vi "frontEnd.vi"(8 "error in (no error)":errorcluster, 11 "ScriptEditorV2 in":refnum<class "ScriptEditorV2.lvclass">) -> (0 "error out":errorcluster, 3 "ScriptEditorV2 out":refnum<class "ScriptEditorV2.lvclass">)   [LabVIEW 2009, in "Views.lvlib" / "ScriptEditor.lvlib" / "ScriptEditorV2.lvclass"]
uses:
  ScriptEditorV2.lvclass
  ScriptEditorV2.lvclass/ScriptEditorV2.ctl
  ScriptEdEvents/ScriptEdEvents.lvclass
  Tools/DatabaseHelpers.lvlib
panel:
  in  "Delete Event":bool
  in  "highlightChannel":bool
  in  "open":bool
  in  "saveAs":bool
  in  "save":bool
  in  "Script Information":string
  out "Multicolumn Listbox":i32[](listbox)
  # "Open"
  # "save"
  # "saveAs"
  # "Highlight"
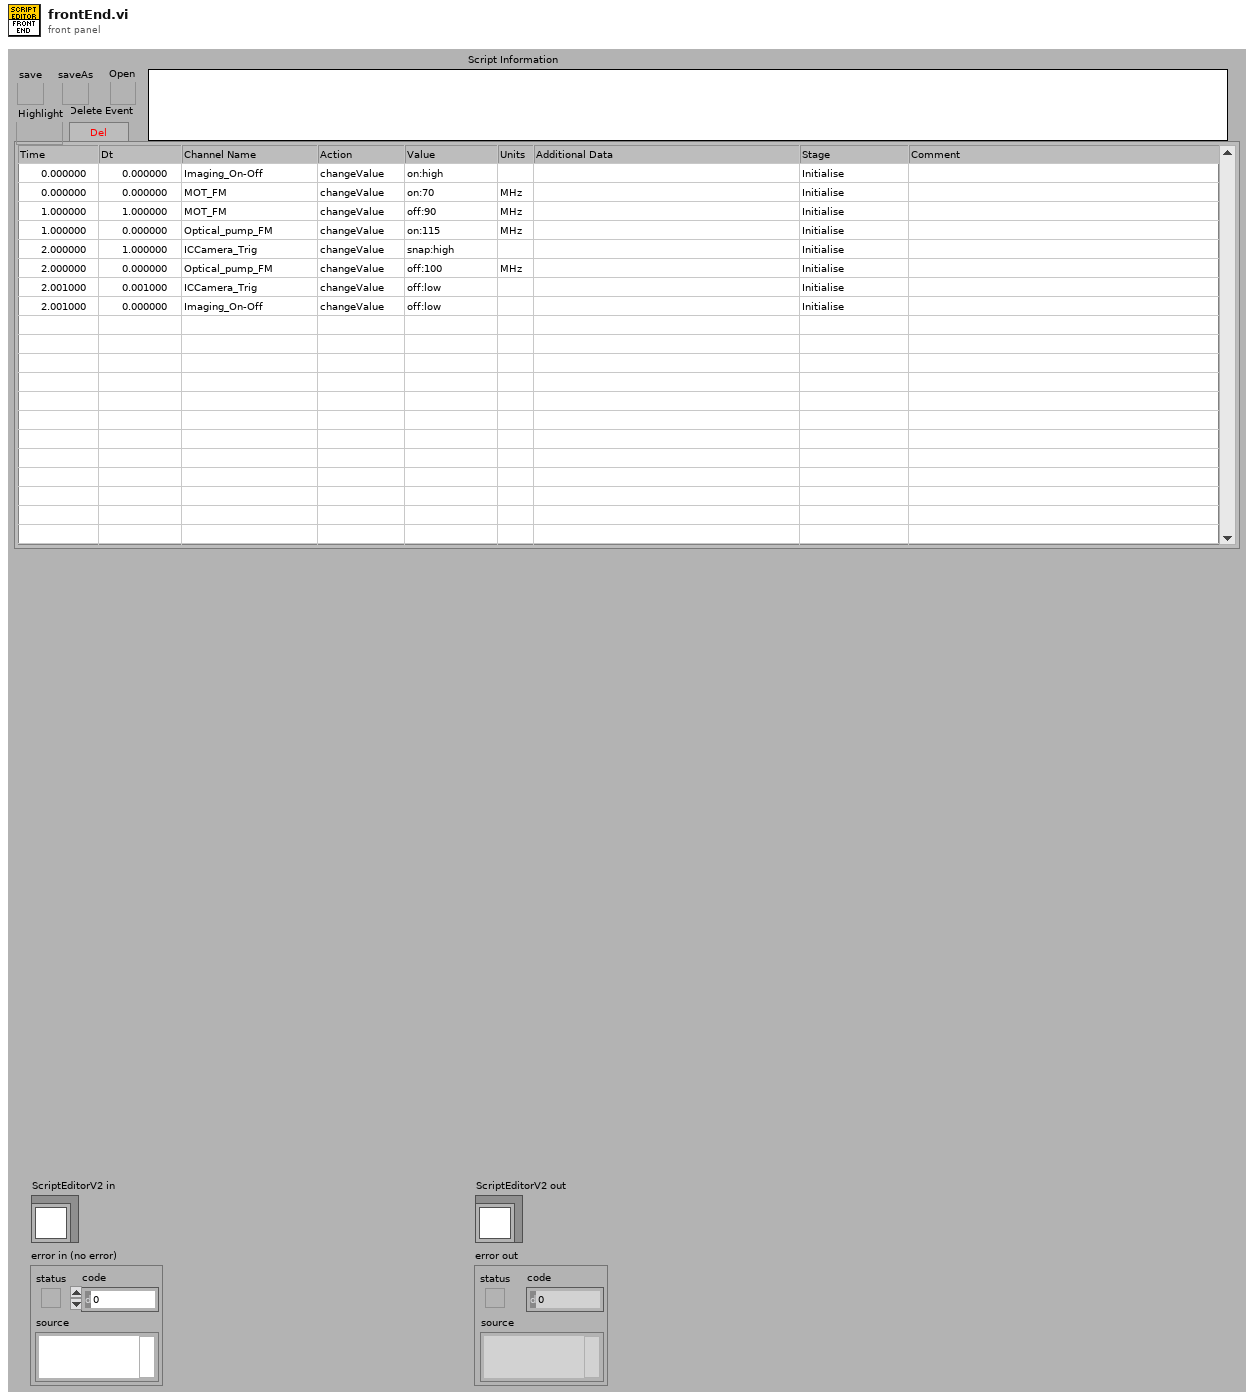
[diagram p1: front panel]
types:
  T1 = typedef "LVPoint32TypeDef.ctl" = cluster{"Horizontal":i32, "Vertical":i32}
  T2 = typedef "LVRowAndColumnTypeDef.ctl" = cluster{"Row":i32, "Column":i32}
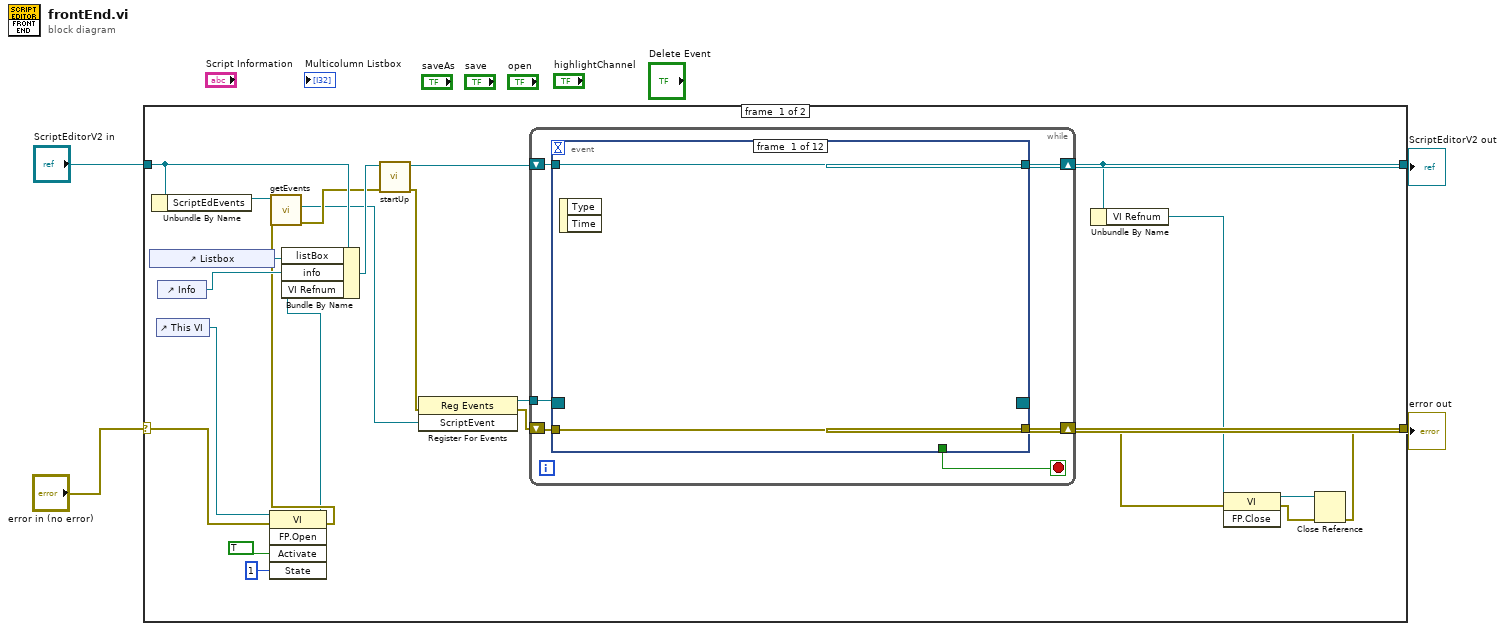
[diagram p0: block diagram]
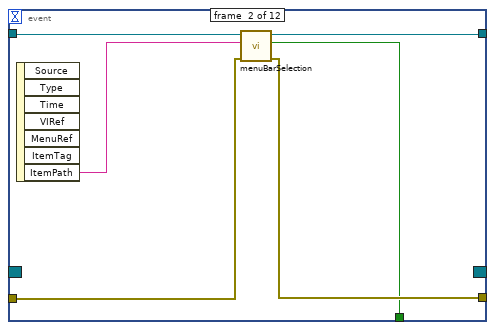
[diagram p2: hidden frame]
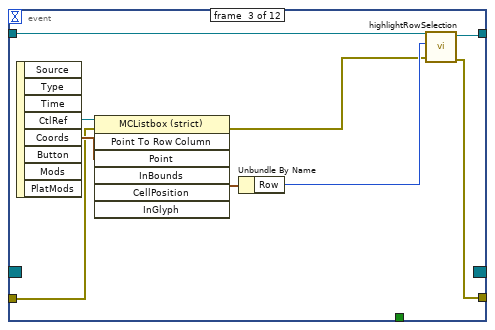
[diagram p3: hidden frame]
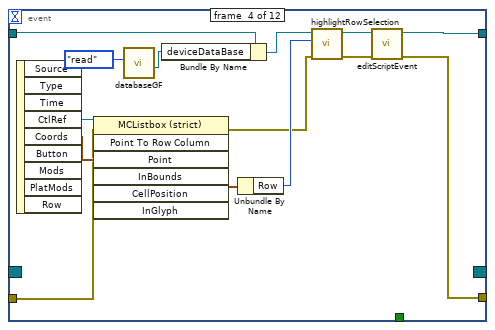
[diagram p4: hidden frame]
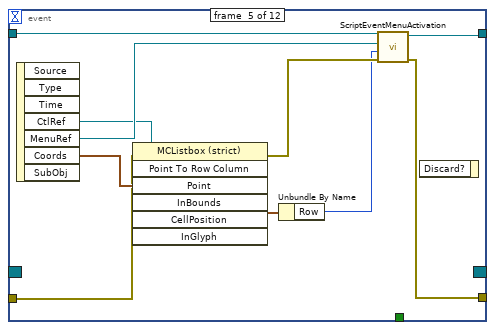
[diagram p5: hidden frame]
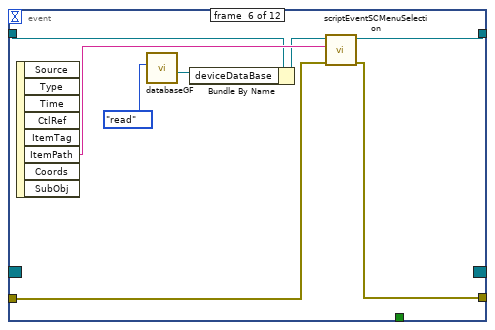
[diagram p6: hidden frame]
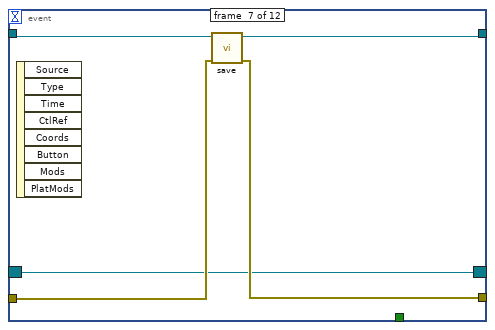
[diagram p7: hidden frame]
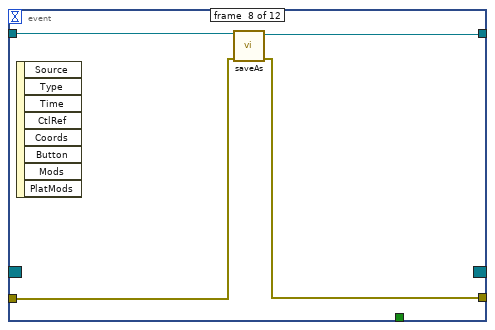
[diagram p8: hidden frame]
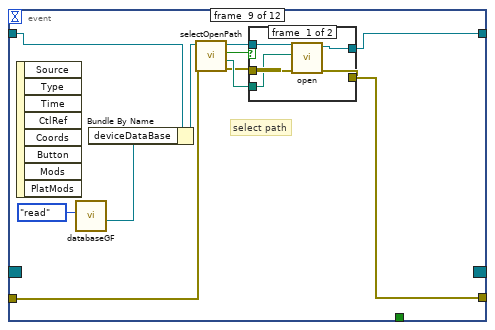
[diagram p9: hidden frame]
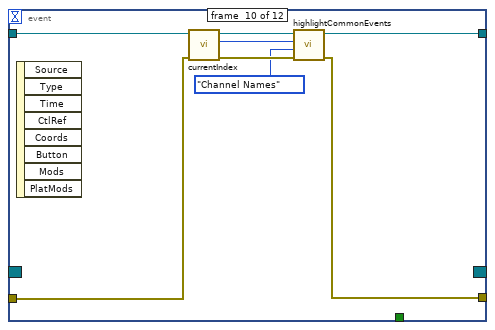
[diagram p11: hidden frame]
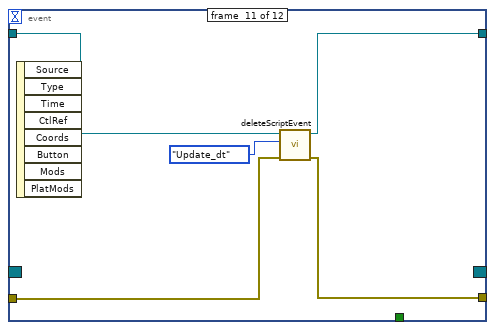
[diagram p12: hidden frame]
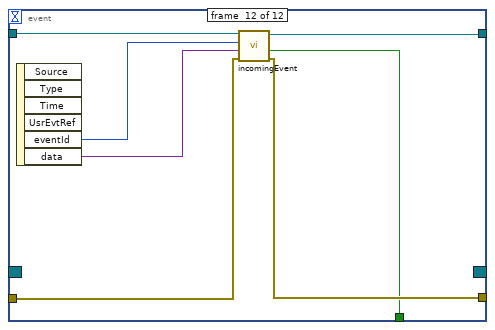
[diagram p13: hidden frame]
diagram:
  n1 = case shown="No Error" "error in (no error)" {
    selector: "error in (no error)" -> [w13 w131]
    tunnel: [w5 w131] -> w3
    tunnel: [w10 w130] -> w1
    tunnel: "ScriptEditorV2 in" -> [w24 w130]
    frame #0 {
      n2 = control-ref of="Listbox"() -> (w17:refnum<vi>)
      n3 = Unbundle By Name(w24) -> ("ScriptEdEvents"=w23:refnum<class "ScriptEdEvents.lvclass">)
      n4 = control-ref of="This VI"() -> (w14:refnum<vi>)
      n5 = control-ref of="Info"() -> (w26:refnum<vi>)
      n6 = invoke class="VI" method="FP.Open"(reference=w14, error in=w13, "Activate"=TRUE, "State"=1) -> (reference out=w11:refnum<vi>, error out=w12:errorcluster)  [unwired: 1 in, 3 out]
      n7 = call-dynamic "getEvents.vi"("error in (no error)"=w12, "ScriptEdEvents in"=w23) -> ("error out"=w21:errorcluster, "ScriptEvent"=w20:refnum<user-event>)  [unwired: 6 in, 2 out]
      n8 = Bundle By Name(cluster=w24, "listBox"=w17, "info"=w26, "VI Refnum"=w11) -> (w25:refnum<class "ScriptEditorV2.lvclass">)
      n9 = call "startUp.vi"("error in (no error)"=w21, "ScriptEditorV2 in"=w25) -> ("error out"=w18:errorcluster, "ScriptEditorV2 out"=w27:refnum<class "ScriptEditorV2.lvclass">)  [unwired: 8 in]
      n10 = register-events(error in=w18, w20) -> (reference out=w22:refnum<event-registration>, error out=w19:errorcluster)  [unwired: 1 in]
      n11 = while {
        shift-right: [w33] -> w10
        shift-left: w27 -> [w28]
        shift-right: [w31] -> w8
        shift-left: w19 -> [w32]
        tunnel: w22 -> [w29]
        stop <- w30 stop-if-true
        n12 = event shown="[2] \"Multicolumn Listbox\": Mouse Down" {
          selector: w29 -> [_ _ _ _ _ _ w83 _ _ _ _ _]
          dyn-events: [_ _ _ _ _ _ w83 _ _ _ _ _] -> _
          timeout: _ -> [_ _ _ _ _ _ _ _ _ _ _ _]
          tunnel: w28 -> [w35 w41 w43 w52 w74 w77 w87 w91 w94 w113 w119 w129]
          tunnel: [w35 w40 w46 w56 w73 w82 w86 w90 w98 w112 w118 w128] -> w33
          tunnel: [w34 w38 w45 w55 w72 w80 w84 w88 w97 w110 w120 w126] -> w31
          tunnel: w32 -> [w34 w39 w48 w61 w68 w81 w85 w89 w96 w111 w121 w127]
          tunnel: [_ w37 _ _ _ _ _ _ _ _ _ w123] -> w30
          event #0 {
            n13 = event-data() -> ()  [unwired: 1 in, 2 out]
          }
          event #1 {
            n14 = event-data() -> ("ItemPath"=w36:string)  [unwired: 1 in, 6 out]
            n15 = call "menuBarSelection.vi"("error in (no error)"=w39, "itemPath"=w36, "ScriptEditorV2 in"=w41) -> ("error out"=w38:errorcluster, "close"=w37:bool, "ScriptEditorV2 out"=w40:refnum<class "ScriptEditorV2.lvclass">)  [unwired: 6 in]
          }
          event #2 {
            n16 = event-data() -> ("CtlRef"=w50:refnum<vi>, "Coords"=w49:T1)  [unwired: 1 in, 6 out]
            n17 = invoke class="MCListbox (strict)" method="Point To Row Column"(reference=w50, error in=w48, "Point"=w49) -> (error out=w42:errorcluster, "CellPosition"=w47:T2)  [unwired: 4 in, 5 out]
            n18 = Unbundle By Name(w47) -> ("Row"=w44:i32)
            n19 = call "highlightRowSelection.vi"("error in (no error)"=w42, "rowIndex"=w44, "ScriptEditorV2 in"=w43) -> ("error out"=w45:errorcluster, "ScriptEditorV2 out"=w46:refnum<class "ScriptEditorV2.lvclass">)  [unwired: 7 in]
          }
          event #3 {
            n20 = event-data() -> ("CtlRef"=w63:refnum<vi>, "Coords"=w62:T1)  [unwired: 1 in, 7 out]
            n21 = invoke class="MCListbox (strict)" method="Point To Row Column"(reference=w63, error in=w61, "Point"=w62) -> (error out=w59:errorcluster, "CellPosition"=w64:T2)  [unwired: 4 in, 5 out]
            n22 = call "databaseGF.vi"("Enum"=enum16{"write", "read"}."read") -> ("deviceDataBase out"=w53:refnum<class "deviceDataBase.lvclass">)  [unwired: 10 in]
            n23 = Bundle By Name(cluster=w52, "deviceDataBase"=w53) -> (w51:refnum<class "ScriptEditorV2.lvclass">)
            n24 = Unbundle By Name(w64) -> ("Row"=w60:i32)
            n25 = call "highlightRowSelection.vi"("error in (no error)"=w59, "rowIndex"=w60, "ScriptEditorV2 in"=w51) -> ("error out"=w57:errorcluster, "ScriptEditorV2 out"=w58:refnum<class "ScriptEditorV2.lvclass">)  [unwired: 7 in]
            n26 = call "editScriptEvent.vi"("error in (no error)"=w57, "ScriptEditorV2 in"=w58) -> ("error out"=w55:errorcluster, "ScriptEditorV2 out"=w56:refnum<class "ScriptEditorV2.lvclass">)  [unwired: 8 in]
          }
          event #4 {
            n27 = event-data() -> ("CtlRef"=w70:refnum<vi>, "MenuRef"=w71:refnum<k9>, "Coords"=w69:T1)  [unwired: 1 in, 4 out]
            n28 = invoke class="MCListbox (strict)" method="Point To Row Column"(reference=w70, error in=w68, "Point"=w69) -> (error out=w66:errorcluster, "CellPosition"=w67:T2)  [unwired: 4 in, 5 out]
            n29 = Unbundle By Name(w67) -> ("Row"=w65:i32)
            n30 = call "ScriptEventMenuActivation.vi"("error in (no error)"=w66, "rowIndex"=w65, "MenuRef"=w71, "ScriptEditorV2 in"=w74) -> ("error out"=w72:errorcluster, "ScriptEditorV2 out"=w73:refnum<class "ScriptEditorV2.lvclass">)  [unwired: 6 in]
            n31 = event-data() -> ()  [unwired: 2 in, 1 out]
          }
          event #5 {
            n32 = event-data() -> ("ItemPath"=w79:string)  [unwired: 1 in, 7 out]
            n33 = call "databaseGF.vi"("Enum"=enum16{"write", "read"}."read") -> ("deviceDataBase out"=w75:refnum<class "deviceDataBase.lvclass">)  [unwired: 10 in]
            n34 = Bundle By Name(cluster=w77, "deviceDataBase"=w75) -> (w76:refnum<class "ScriptEditorV2.lvclass">)
            n35 = call "scriptEventSCMenuSelection.vi"("error in (no error)"=w81, "path"=w79, "ScriptEditorV2 in"=w76) -> ("error out"=w80:errorcluster, "ScriptEditorV2 out"=w82:refnum<class "ScriptEditorV2.lvclass">)  [unwired: 7 in]
          }
          event #6 {
            n36 = event-data() -> ()  [unwired: 1 in, 8 out]
            n37 = call "save.vi"("error in (no error)"=w85, "ScriptEditorV2 in"=w87) -> ("error out"=w84:errorcluster, "ScriptEditorV2 out"=w86:refnum<class "ScriptEditorV2.lvclass">)  [unwired: 8 in]
          }
          event #7 {
            n38 = event-data() -> ()  [unwired: 1 in, 8 out]
            n39 = call "saveAs.vi"("error in (no error)"=w89, "ScriptEditorV2 in"=w91) -> ("error out"=w88:errorcluster, "ScriptEditorV2 out"=w90:refnum<class "ScriptEditorV2.lvclass">)  [unwired: 8 in]
          }
          event #8 {
            # "select path"
            n40 = event-data() -> ()  [unwired: 1 in, 8 out]
            n41 = call "databaseGF.vi"("Enum"=enum16{"write", "read"}."read") -> ("deviceDataBase out"=w92:refnum<class "deviceDataBase.lvclass">)  [unwired: 10 in]
            n42 = Bundle By Name(cluster=w94, "deviceDataBase"=w92) -> (w93:refnum<class "ScriptEditorV2.lvclass">)
            n43 = call "selectOpenPath.vi"("error in (no error)"=w96, "ScriptEditorV2 in"=w93) -> ("error out"=w99:errorcluster, "selected path"=w101:path, "notSelected?"=w100:bool, "ScriptEditorV2 out"=w102:refnum<class "ScriptEditorV2.lvclass">)  [unwired: 6 in]
            n44 = case shown="False" w100 {
              tunnel: [w107 w109] -> w98
              tunnel: w99 -> [w106 w108]
              tunnel: [w105 w108] -> w97
              tunnel: w102 -> [w104 w109]
              tunnel: w101 -> [w103 _]
              frame #0 {
                n45 = call "open.vi"("error in (no error)"=w106, "Path"=w103, "ScriptEditorV2 in"=w104) -> ("error out"=w105:errorcluster, "ScriptEditorV2 out"=w107:refnum<class "ScriptEditorV2.lvclass">)  [unwired: 7 in]
              }
              frame #1 {
              }
            }
          }
          event #9 {
            n46 = event-data() -> ()  [unwired: 1 in, 8 out]
            n47 = call "currentIndex.vi"("error in (no error)"=w111, "ScriptEditorV2 in"=w113) -> ("error out"=w116:errorcluster, "index"=w117:i32, "ScriptEditorV2 out"=w115:refnum<class "ScriptEditorV2.lvclass">)  [unwired: 7 in]
            n48 = call "highlightCommonEvents.vi"("error in (no error)"=w116, "Enum"=enum16{"Channel Names", "Stage"}."Channel Names", "rowIndex"=w117, "ScriptEditorV2 in"=w115) -> ("error out"=w110:errorcluster, "ScriptEditorV2 out"=w112:refnum<class "ScriptEditorV2.lvclass">)  [unwired: 6 in]
          }
          event #10 {
            n49 = event-data() -> ()  [unwired: 1 in, 8 out]
            n50 = call "deleteScriptEvent.vi"("error in (no error)"=w121, "Enum"=enum16{"Update_dt", "Update_Time"}."Update_dt", "ScriptEditorV2 in"=w119) -> ("error out"=w120:errorcluster, "ScriptEditorV2 out"=w118:refnum<class "ScriptEditorV2.lvclass">)  [unwired: 7 in]
          }
          event #11 {
            n51 = event-data() -> ("eventId"=w125:enum16{"Open", "Save", "Close"}, "data"=w124:variant)  [unwired: 1 in, 4 out]
            n52 = call "incomingEvent.vi"("error in (no error)"=w127, "data"=w124, "eventId"=w125, "ScriptEditorV2 in"=w129) -> ("error out"=w126:errorcluster, "close"=w123:bool, "ScriptEditorV2 out"=w128:refnum<class "ScriptEditorV2.lvclass">)  [unwired: 5 in]
          }
        }
      }
      n53 = Unbundle By Name(w10) -> ("VI Refnum"=w9:refnum<vi>)
      n54 = invoke class="VI" method="FP.Close"(reference=w9, error in=w8) -> (reference out=w6:refnum<vi>, error out=w7:errorcluster)  [unwired: 1 in, 1 out]
      n55 = Close Reference(reference=w6, error in (no error)=w7) -> (error out=w5:errorcluster)
    }
    frame #1 {
    }
  }
  "error out" <- w3
  "ScriptEditorV2 out" <- w1
